vi "Fill Out 3rd Party VIs .vi"(7 "3rd Party Member Data":string[][](array[string]), 8 "error in (no error)":errorcluster, 11 "NI_report in":refnum<class "NI_report.lvclass">) -> (0 "error out":errorcluster, 3 "NI_report out":refnum<class "NI_report.lvclass">)   [LabVIEW 2014]
uses:
  <vilib>/Utility/NIReport.llb/NI_report.lvclass
  <vilib>/addons/_office/excel.llb/Excel Easy Table (str).vi
  <vilib>/Utility/NIReport.llb/Excel/NI_Excel.lvclass
  <vilib>/addons/_office/NI_ReportGenerationToolkit.lvlib
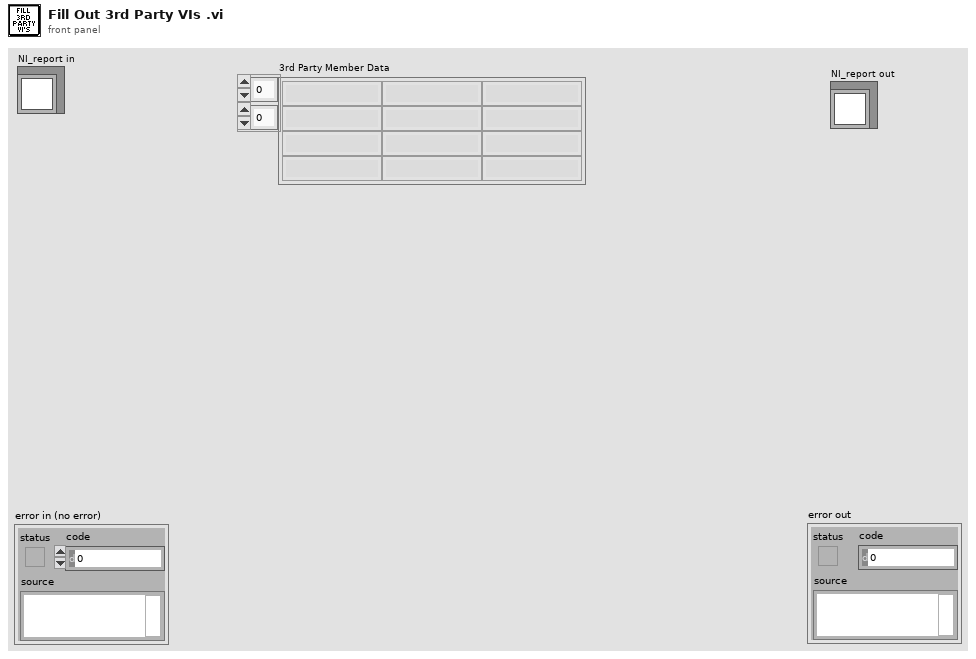
[diagram p1: front panel]
types:
  T1 = cluster{"on/off":bool, "weight":i32, "color":u32}
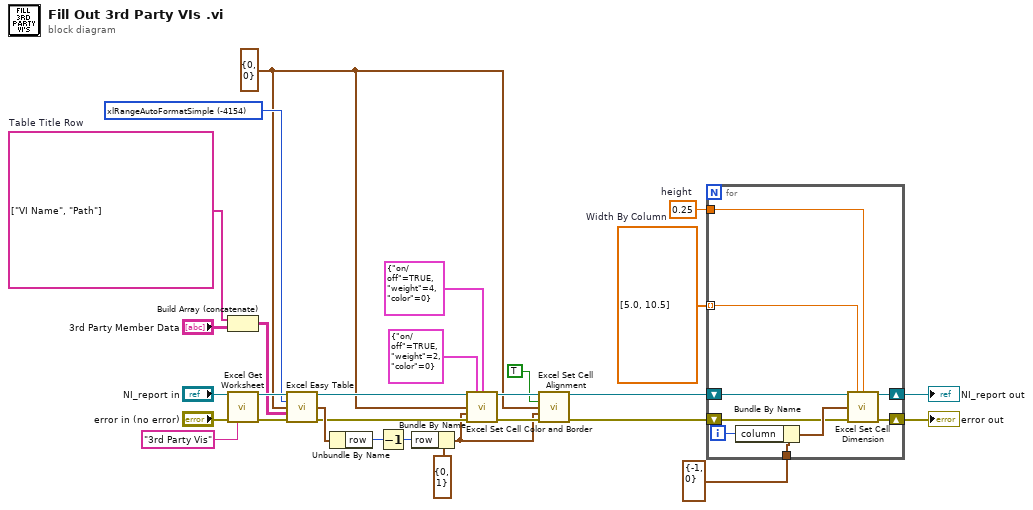
[diagram p0: block diagram]
diagram:
  w8 = 0.25  # height
  w13 = dbl[] [5.0, 10.5]  # Width By Column
  w20 = string[] ["VI Name", "Path"]  # Table Title Row
  w21 = -4154 items=["xlRangeAutoFormat3DEffects1"=13, "xlRangeAutoFormat3DEffects2"=14, "xlRangeAutoFormatAccounting1"=4, "xlRangeAutoFormatAccounting2"=5, "xlRangeAutoFormatAccounting3"=6, "xlRangeAutoFormatAccounting4"=17, "xlRangeAutoFormatClassic1"=1, "xlRangeAutoFormatClassic2"=2, "xlRangeAutoFormatClassic3"=3, "xlRangeAutoFormatColor1"=7, "xlRangeAutoFormatColor2"=8, "xlRangeAutoFormatColor3"=9, "xlRangeAutoFormatList1"=10, "xlRangeAutoFormatList2"=11, "xlRangeAutoFormatList3"=12, "xlRangeAutoFormatLocalFormat1"=15, "xlRangeAutoFormatLocalFormat2"=16, "xlRangeAutoFormatLocalFormat3"=19, "xlRangeAutoFormatLocalFormat4"=20, "xlRangeAutoFormatReport1"=21, "xlRangeAutoFormatReport2"=22, "xlRangeAutoFormatReport3"=23, "xlRangeAutoFormatReport4"=24, "xlRangeAutoFormatReport5"=25, "xlRangeAutoFormatReport6"=26, "xlRangeAutoFormatReport7"=27, "xlRangeAutoFormatReport8"=28, "xlRangeAutoFormatReport9"=29, "xlRangeAutoFormatReport10"=30, "xlRangeAutoFormatClassicPivotTable"=31, "xlRangeAutoFormatTable1"=32, "xlRangeAutoFormatTable2"=33, "xlRangeAutoFormatTable3"=34, "xlRangeAutoFormatTable4"=35, "xlRangeAutoFormatTable5"=36, "xlRangeAutoFormatTable6"=37, "xlRangeAutoFormatTable7"=38, "xlRangeAutoFormatTable8"=39, "xlRangeAutoFormatTable9"=40, "xlRangeAutoFormatTable10"=41, "xlRangeAutoFormatPTNone"=42, "xlRangeAutoFormatNone"=-4142, "xlRangeAutoFormatSimple"=-4154] ("auto format (none)")
  w12 = cluster{"row":i32, "column":i32} {"row"=0, "column"=0} ("start (-1, -1)")
  n1 = Build Array (concatenate)(w20, "3rd Party Member Data") -> (w18:string[][])
  n2 = call <vilib>:"Excel Get Worksheet.vi"("report in"="NI_report in", "error in (no error)"="error in (no error)", "name (\"\")"="3rd Party Vis" ("name (\"\")")) -> ("report out"=w26:refnum<class "NI_report.lvclass">, "error out"=w27:errorcluster)  [unwired: 11 in]
  n3 = call-poly <vilib>:"Excel Easy Table.vi"("report in"=w26, "auto format (none)"=w21, "start (0, 0)"=w12, "text data"=w18, "error in (no error)"=w27) -> ("report out"=w24:refnum<class "NI_report.lvclass">, "next cell bottom-left"=w16:cluster{"row":i32, "column":i32}, "error out"=w10:errorcluster)  [unwired: 6 in, 2 out]
  n4 = Unbundle By Name(w16) -> ("row"=w3:i32)
  n5 = Decrement(x=w3) -> (x-1=w15:i32)
  n6 = Bundle By Name(cluster=cluster{"row":i32, "column":i32} {"row"=0, "column"=1} ("start (-1, -1)"), "row"=w15) -> (w5:cluster{"row":i32, "column":i32})
  n7 = call <vilib>:"Excel Set Cell Color and Border.vi"("report in"=w24, "inside border"=T1 {"on/off"=TRUE, "weight"=2, "color"=0}, "outside border"=T1 {"on/off"=TRUE, "weight"=4, "color"=0}, "start (-1, -1)"=w12, "end (-1, -1)"=w5, "error in (no error)"=w10) -> ("report out"=w17:refnum<class "NI_report.lvclass">, "error out"=w9:errorcluster)  [unwired: 8 in]
  n8 = call <vilib>:"Excel Set Cell Alignment.vi"("report in"=w17, "wrap text? (F)"=TRUE, "start (-1, -1)"=w12, "end (-1, -1)"=w5, "error in (no error)"=w9) -> ("report out"=w7:refnum<class "NI_report.lvclass">, "error out"=w6:errorcluster)  [unwired: 9 in]
  n9 = for {
    tunnel: w13 -> [w36] mode=indexing
    tunnel: cluster{"row":i32, "column":i32} {"row"=-1, "column"=0} ("start (-1, -1)") -> [w35]
    shift-right: [w37] -> w2
    shift-left: w7 -> [w38]
    shift-right: [w34] -> w1
    shift-left: w6 -> [w31]
    tunnel: w8 -> [w30]
    i -> [w32]
    n10 = Bundle By Name(cluster=w35, "column"=w32) -> (w33:cluster{"row":i32, "column":i32})
    n11 = call <vilib>:"Excel Set Cell Dimension.vi"("report in"=w38, "width (-1)"=w36, "height (-1)"=w30, "start (-1, -1)"=w33, "error in (no error)"=w31) -> ("report out"=w37:refnum<class "NI_report.lvclass">, "error out"=w34:errorcluster)  [unwired: 9 in]
  }
  "error out" <- w1
  "NI_report out" <- w2
